vi "Configure Thermocouple.vi"(0 "VISA resource name":refnum<visa-resource-name>, 1 "Thermocouple Type (0: J)":u16(ring) items=["J", "K", "T"], 2 "R-Junction Type (0: Simulated)":u16(ring) items=["Simulated", "Real"], 5 "error in (no error)":errorcluster, 6 "Simulated Temperature (23.00 deg)":dbl=23.0 format="%_4f", 8 "Temperature Coefficient (2.00E-4 deg C/V)":dbl=0.0002 format="%_3e", 10 "Voltage Offset (5.463E-2 V)":dbl=0.05463 format="%_4e") -> (14 "VISA resource name out":refnum<visa-resource-name>, 19 "error out":errorcluster)   [LabVIEW 2016, in "Keithley 2000.lvlib"]
doc: "This VI configures the thermocouple type and settings."
uses:
  Keithley 2000.lvlib
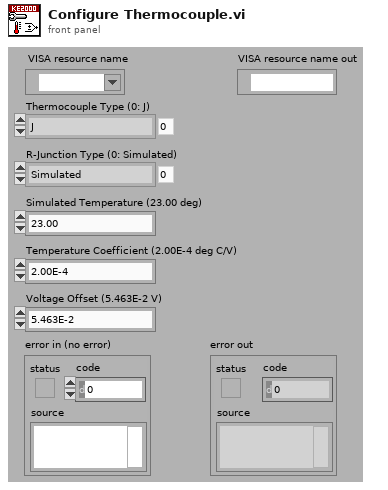
[diagram p1: front panel]
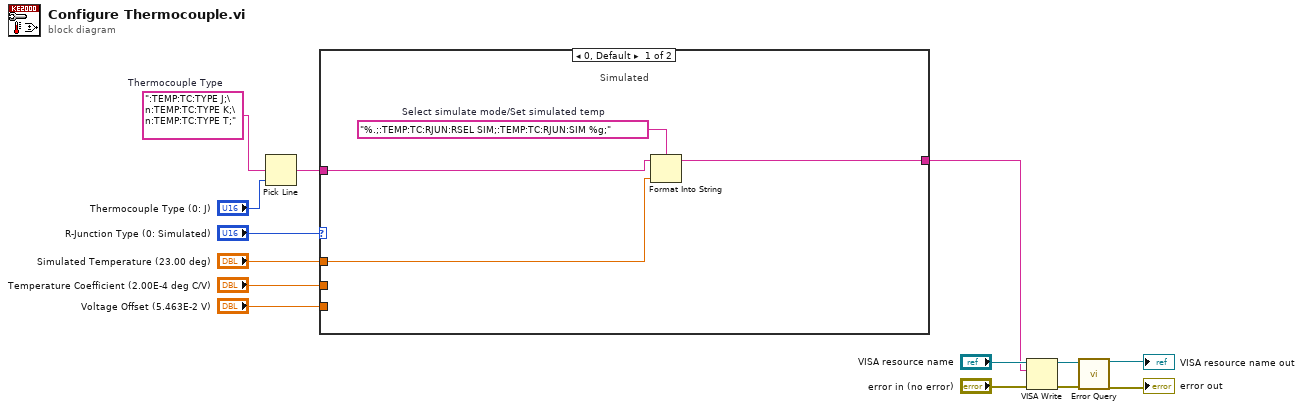
[diagram p0: block diagram]
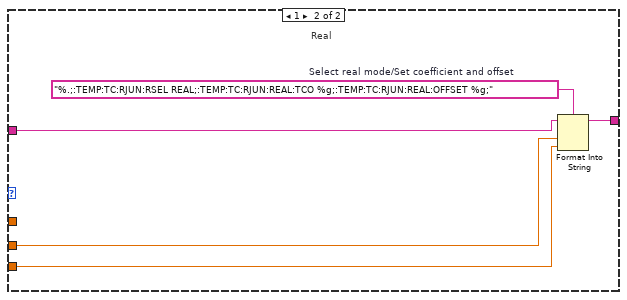
[diagram p2: hidden frame]
diagram:
  w12 = ":TEMP:TC:TYPE J;\n:TEMP:TC:TYPE K;\n:TEMP:TC:TYPE T;"  # Thermocouple Type
  n1 = Pick Line(multi-line string=w12, line index="Thermocouple Type (0: J)") -> (output string=w6:string)  [unwired: 1 in]
  n2 = case shown="0, Default" "R-Junction Type (0: Simulated)" {
    tunnel: "Simulated Temperature (23.00 deg)" -> [w16 _]
    tunnel: "Temperature Coefficient (2.00E-4 deg C/V)" -> [_ w21]
    tunnel: "Voltage Offset (5.463E-2 V)" -> [_ w20]
    tunnel: w6 -> [w18 w23]
    tunnel: [w15 w19] -> w5
    frame 0, Default {
      w17 = "%.;:TEMP:TC:RJUN:RSEL SIM;:TEMP:TC:RJUN:SIM %g;"  # Select simulate mode/Set simulated temp
      # "Simulated"
      n3 = Format Into String(format string=w17, initial string=w18, w16) -> (resulting string=w15:string)  [unwired: 1 in, 1 out]
    }
    frame 1 {
      w22 = "%.;:TEMP:TC:RJUN:RSEL REAL;:TEMP:TC:RJUN:REAL:TCO %g;:TEMP:TC:RJUN:REAL:OFFSET %g;"  # Select real mode/Set coefficient and offset
      # "Real"
      n4 = Format Into String(format string=w22, initial string=w23, w21, w20) -> (resulting string=w19:string)  [unwired: 1 in, 1 out]
    }
  }
  n5 = VISA Write(VISA resource name="VISA resource name", write buffer=w5, error in (no error)="error in (no error)") -> (VISA resource name out=w4:refnum<visa-resource-name>, error out=w2:errorcluster)  [unwired: 1 out]
  n6 = call "Error Query.vi"("VISA resource name"=w4, "error in (no error)"=w2) -> ("VISA resource name out"=→"VISA resource name out":refnum<visa-resource-name>, "error out"=→"error out":errorcluster)  [unwired: 14 in, 2 out]
